vi "Data Logging_Generate Data String.vi"(8 "error in":errorcluster, 10 "Measurement Data":T1, 11 "Data Logging Options":T2={"Absolute Press."=TRUE, "Gauge/Diff. Press."=TRUE, "Barometric Press."=TRUE, "Temperature"=TRUE, "Volumetric"=TRUE, "Mass Flow"=TRUE, "Setpoint"=TRUE, "Valve Drive"=FALSE, "Totalizer"=TRUE, "Tot. Timer [s]"=FALSE, "Tot. Avg. Flow"=FALSE, "Tot. Peak Flow"=FALSE, "Gas Selected"=TRUE, "Log Data"=FALSE}) -> (0 "error out":errorcluster, 2 "Log Data":bool, 3 "Data Log String":string)   [LabVIEW 2014]
doc: "Generates a comma delimited string from the data based on the logging options selected. This is for use with LabVIEW's \"Write to Text File\" sub-VI to make data logging easier."
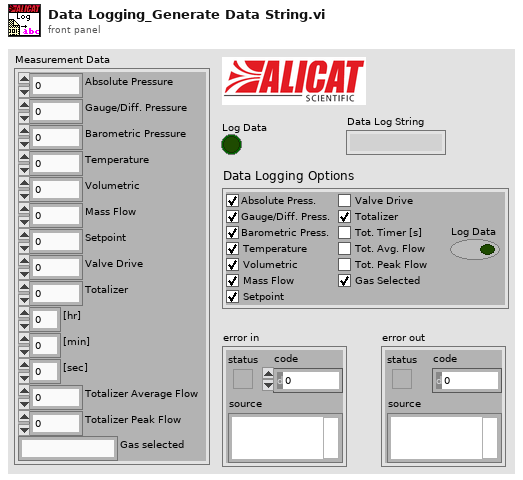
[diagram p1: front panel]
types:
  T1 = cluster{"Absolute Pressure":dbl, "Gauge/Diff. Pressure":dbl, "Barometric Pressure":dbl, "Temperature":dbl, "Volumetric":dbl, "Mass Flow":dbl, "Setpoint":dbl, "Valve Drive":dbl, "Totalizer":dbl, "[hr]":dbl, "[min]":dbl, "[sec]":dbl, "Totalizer Average Flow":dbl, "Totalizer Peak Flow":dbl, "Gas selected":string}
  T2 = cluster{"Absolute Press.":bool, "Gauge/Diff. Press.":bool, "Barometric Press.":bool, "Temperature":bool, "Volumetric":bool, "Mass Flow":bool, "Setpoint":bool, "Valve Drive":bool, "Totalizer":bool, "Tot. Timer [s]":bool, "Tot. Avg. Flow":bool, "Tot. Peak Flow":bool, "Gas Selected":bool, "Log Data":bool}
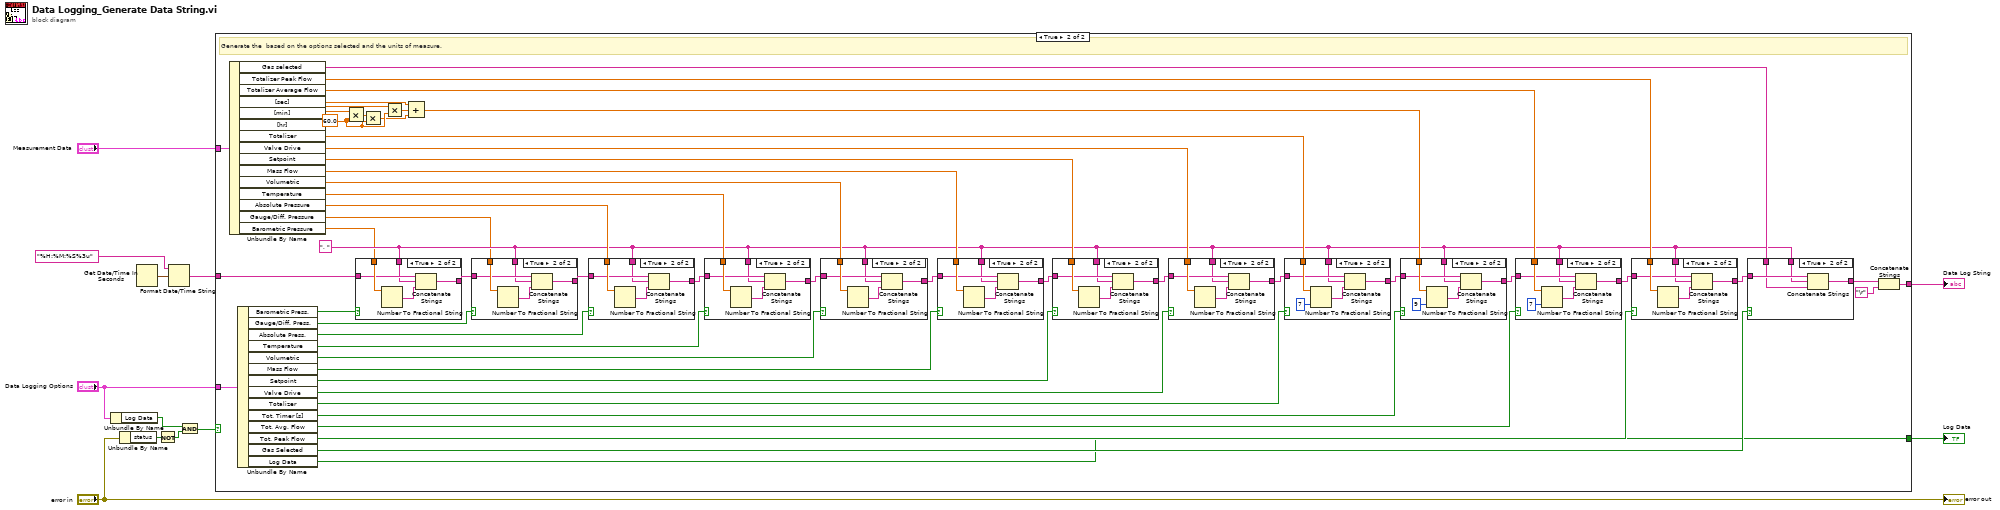
[diagram p0: block diagram]
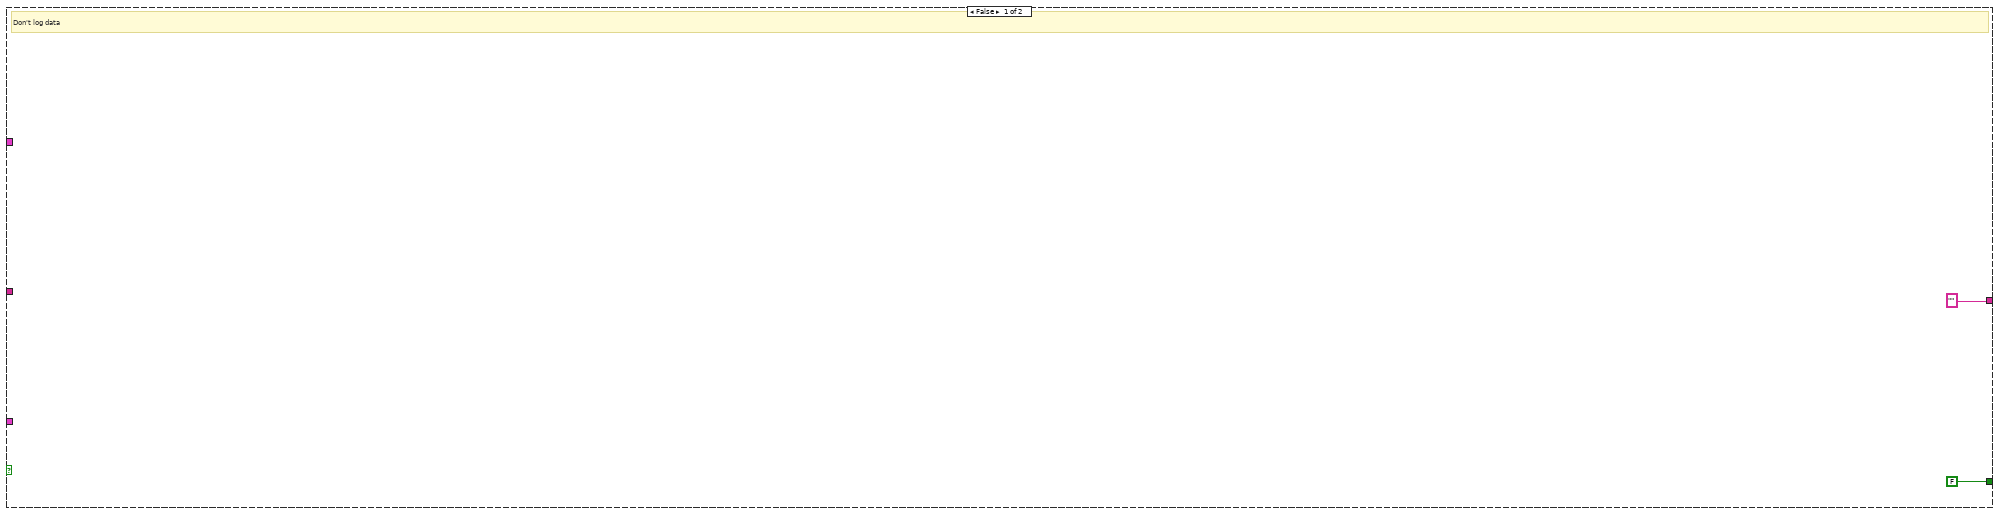
[diagram p2: hidden frame]
diagram:
  n1 = Unbundle By Name("Data Logging Options") -> ("Log Data"=w11:bool)
  n2 = Unbundle By Name("error in") -> ("status"=w5:bool)
  n3 = Get Date/Time In Seconds() -> (seconds since 1Jan1904=w7:timestamp)
  n4 = Not(x=w5) -> (.not. x?=w4:bool)
  n5 = Format Date/Time String(time format string (%c)="%H:%M:%S%3u", seconds (now)=w7) -> (date/time string=w6:string)  [unwired: 1 in]
  n6 = And(x=w11, y=w4) -> (x .and. y?=w10:bool)
  n7 = case shown="True" w10 {
    tunnel: "Data Logging Options" -> [_ w66]
    tunnel: ["" ("string") w24] -> w12
    tunnel: "Measurement Data" -> [_ w65]
    tunnel: w6 -> [_ w21]
    tunnel: [FALSE ("Log Data") w23] -> w3
    frame False {
      # "Don't log data"
    }
    frame True {
      w61 = 60.0 ("y")
      w17 = ", " ("string")
      # "Generate the  based on the options selected and the units of measure."
      n8 = Unbundle By Name(w65) -> ("Gas selected"=w27:string, "Totalizer Peak Flow"=w28:dbl, "Totalizer Average Flow"=w29:dbl, "[sec]"=w60:dbl, "[min]"=w62:dbl, "[hr]"=w63:dbl, "Totalizer"=w31:dbl, "Valve Drive"=w32:dbl, "Setpoint"=w33:dbl, "Mass Flow"=w34:dbl, "Volumetric"=w35:dbl, "Temperature"=w36:dbl, "Absolute Pressure"=w57:dbl, "Gauge/Diff. Pressure"=w16:dbl, "Barometric Pressure"=w15:dbl)
      n9 = Unbundle By Name(w66) -> ("Barometric Press."=w19:bool, "Gauge/Diff. Press."=w18:bool, "Absolute Press."=w67:bool, "Temperature"=w46:bool, "Volumetric"=w45:bool, "Mass Flow"=w44:bool, "Setpoint"=w43:bool, "Valve Drive"=w42:bool, "Totalizer"=w41:bool, "Tot. Timer [s]"=w40:bool, "Tot. Avg. Flow"=w39:bool, "Tot. Peak Flow"=w38:bool, "Gas Selected"=w37:bool, "Log Data"=w23:bool)
      n10 = Multiply(x=w63, y=w61) -> (x*y=w64:dbl)
      n11 = case shown="True" w19 {
        tunnel: w21 -> [w68 w72]
        tunnel: [w68 w69] -> w22
        tunnel: w17 -> [_ w71]
        tunnel: w15 -> [_ w73]
        frame False {
        }
        frame True {
          n12 = Number To Fractional String(number=w73) -> (F-format string=w70:string)  [unwired: 3 in]
          n13 = Concatenate Strings(w72, w71, w70) -> (w69:string)
        }
      }
      n14 = Multiply(x=w64, y=w61) -> (x*y=w58:dbl)
      n15 = Multiply(x=w62, y=w61) -> (x*y=w59:dbl)
      n16 = Compound Arithmetic op=ADD(w60, w59, w58) -> (w30:dbl)
      n17 = case shown="True" w18 {
        tunnel: w22 -> [w74 w78]
        tunnel: [w74 w75] -> w20
        tunnel: w17 -> [_ w77]
        tunnel: w16 -> [_ w79]
        frame False {
        }
        frame True {
          n18 = Number To Fractional String(number=w79) -> (F-format string=w76:string)  [unwired: 3 in]
          n19 = Concatenate Strings(w78, w77, w76) -> (w75:string)
        }
      }
      n20 = case shown="True" w67 {
        tunnel: w20 -> [w142 w146]
        tunnel: [w142 w143] -> w56
        tunnel: w17 -> [_ w145]
        tunnel: w57 -> [_ w147]
        frame False {
        }
        frame True {
          n21 = Number To Fractional String(number=w147) -> (F-format string=w144:string)  [unwired: 3 in]
          n22 = Concatenate Strings(w146, w145, w144) -> (w143:string)
        }
      }
      n23 = case shown="True" w46 {
        tunnel: w56 -> [w136 w140]
        tunnel: [w136 w137] -> w55
        tunnel: w17 -> [_ w139]
        tunnel: w36 -> [_ w141]
        frame False {
        }
        frame True {
          n24 = Number To Fractional String(number=w141) -> (F-format string=w138:string)  [unwired: 3 in]
          n25 = Concatenate Strings(w140, w139, w138) -> (w137:string)
        }
      }
      n26 = case shown="True" w45 {
        tunnel: w55 -> [w130 w134]
        tunnel: [w130 w131] -> w54
        tunnel: w17 -> [_ w133]
        tunnel: w35 -> [_ w135]
        frame False {
        }
        frame True {
          n27 = Number To Fractional String(number=w135) -> (F-format string=w132:string)  [unwired: 3 in]
          n28 = Concatenate Strings(w134, w133, w132) -> (w131:string)
        }
      }
      n29 = case shown="True" w44 {
        tunnel: w54 -> [w124 w128]
        tunnel: [w124 w125] -> w53
        tunnel: w17 -> [_ w127]
        tunnel: w34 -> [_ w129]
        frame False {
        }
        frame True {
          n30 = Number To Fractional String(number=w129) -> (F-format string=w126:string)  [unwired: 3 in]
          n31 = Concatenate Strings(w128, w127, w126) -> (w125:string)
        }
      }
      n32 = case shown="True" w43 {
        tunnel: w53 -> [w118 w122]
        tunnel: [w118 w119] -> w52
        tunnel: w17 -> [_ w121]
        tunnel: w33 -> [_ w123]
        frame False {
        }
        frame True {
          n33 = Number To Fractional String(number=w123) -> (F-format string=w120:string)  [unwired: 3 in]
          n34 = Concatenate Strings(w122, w121, w120) -> (w119:string)
        }
      }
      n35 = case shown="True" w42 {
        tunnel: w52 -> [w112 w116]
        tunnel: [w112 w113] -> w51
        tunnel: w17 -> [_ w115]
        tunnel: w32 -> [_ w117]
        frame False {
        }
        frame True {
          n36 = Number To Fractional String(number=w117) -> (F-format string=w114:string)  [unwired: 3 in]
          n37 = Concatenate Strings(w116, w115, w114) -> (w113:string)
        }
      }
      n38 = case shown="True" w41 {
        tunnel: w51 -> [w105 w110]
        tunnel: [w105 w107] -> w50
        tunnel: w17 -> [_ w109]
        tunnel: w31 -> [_ w111]
        frame False {
        }
        frame True {
          n39 = Number To Fractional String(number=w111, precision (6)=i16 7) -> (F-format string=w108:string)  [unwired: 2 in]
          n40 = Concatenate Strings(w110, w109, w108) -> (w107:string)
        }
      }
      n41 = case shown="True" w40 {
        tunnel: w50 -> [w98 w103]
        tunnel: [w98 w100] -> w49
        tunnel: w17 -> [_ w102]
        tunnel: w30 -> [_ w104]
        frame False {
        }
        frame True {
          n42 = Number To Fractional String(number=w104, precision (6)=i16 9) -> (F-format string=w101:string)  [unwired: 2 in]
          n43 = Concatenate Strings(w103, w102, w101) -> (w100:string)
        }
      }
      n44 = case shown="True" w39 {
        tunnel: w49 -> [w91 w96]
        tunnel: [w91 w93] -> w48
        tunnel: w17 -> [_ w95]
        tunnel: w29 -> [_ w97]
        frame False {
        }
        frame True {
          n45 = Number To Fractional String(number=w97, precision (6)=i16 7) -> (F-format string=w94:string)  [unwired: 2 in]
          n46 = Concatenate Strings(w96, w95, w94) -> (w93:string)
        }
      }
      n47 = case shown="True" w38 {
        tunnel: w48 -> [w85 w89]
        tunnel: [w85 w86] -> w47
        tunnel: w17 -> [_ w88]
        tunnel: w28 -> [_ w90]
        frame False {
        }
        frame True {
          n48 = Number To Fractional String(number=w90) -> (F-format string=w87:string)  [unwired: 3 in]
          n49 = Concatenate Strings(w89, w88, w87) -> (w86:string)
        }
      }
      n50 = case shown="True" w37 {
        tunnel: w47 -> [w80 w84]
        tunnel: [w80 w82] -> w26
        tunnel: w17 -> [_ w83]
        tunnel: w27 -> [_ w81]
        frame False {
        }
        frame True {
          n51 = Concatenate Strings(w84, w83, w81) -> (w82:string)
        }
      }
      n52 = Concatenate Strings(w26, "\r" ("string")) -> (w24:string)
    }
  }
  "Data Log String" <- w12
  "Log Data" <- w3
  "error out" <- "error in"
